vi "Compare file size of FTP to Dir on local Machine.vi"(8 "File Pattern (*.CSV .ddf)":string, 9 "Local Path to compare file sizes to FTP":path, 11 "FTP Creds":T1 {"FTP Timeout (S)" min=0 max=300 step=1}) -> (3 "Equal File Sizes":cluster{"name":string, "Equal File size":bool}[](array[cluster]))   [LabVIEW 2011]
uses:
  Controls/FTP Credintials.ctl
  <vilib>/addons/internet/NI_InternetTK_FTP_VIs.lvlib
panel:
  in  "Archive Location":path=path "C:/Archive" caption="Directory To Archive *.RAT files"
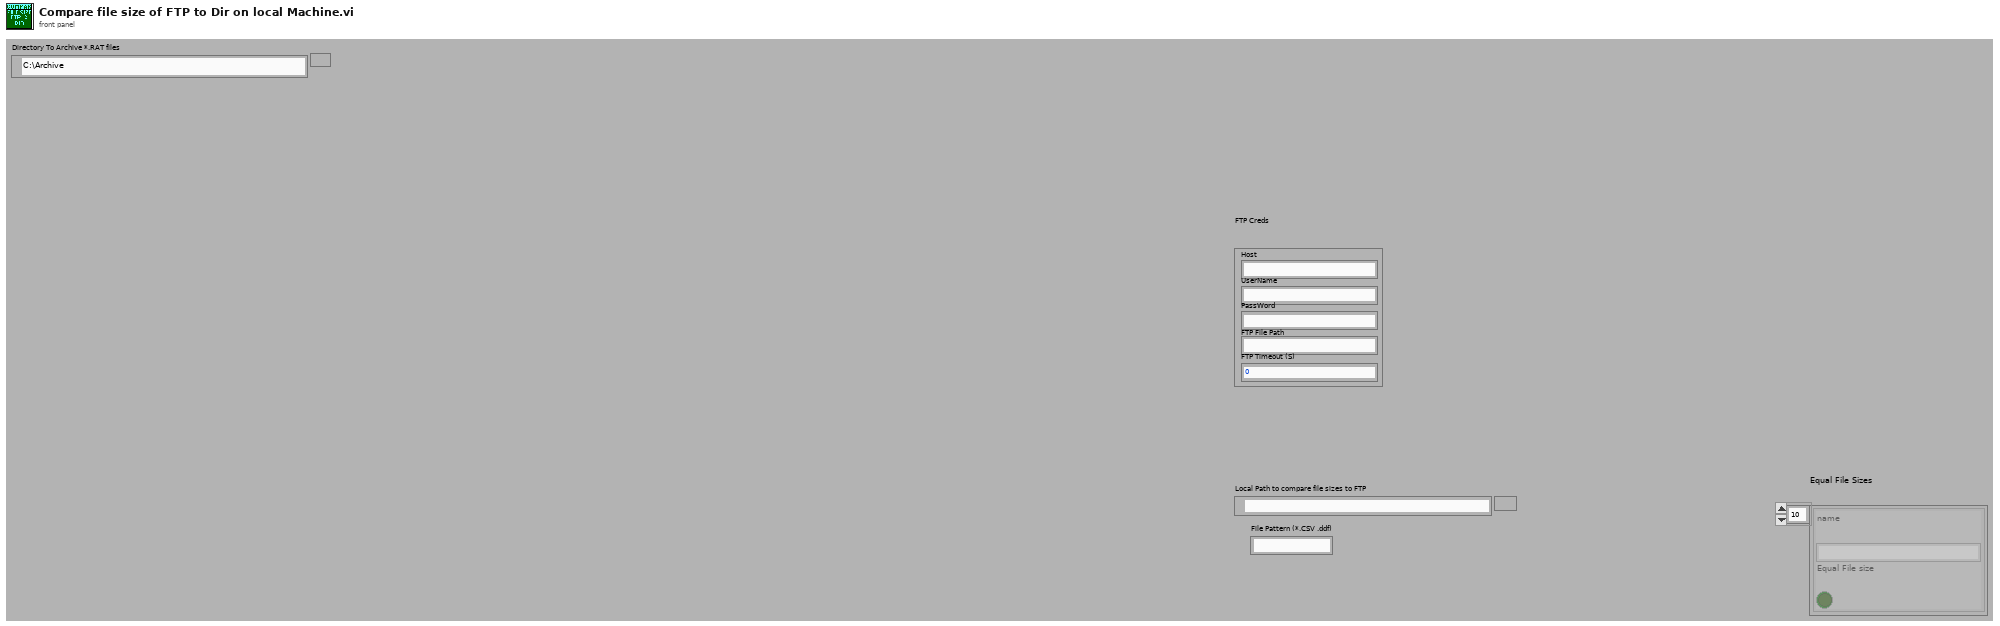
[diagram p1: front panel]
types:
  T1 = typedef "FTP Credintials.ctl" = cluster{"Host":string, "UserName":string, "PassWord":string, "FTP File Path":string, "FTP Timeout (S)":i32, "Active or Passive":bool, "ASCII or Binary":bool}
  T2 = typedef "FTP Session.ctl" = refnum<k1>
  T3 = typedef "FTP File Info.ctl" = cluster{"type":enum16{"unknown", "file", "dir", "link"}, "permissions":string, "owner":string, "group":string, "size":i32, "date":string, "name":string, "link name":string}
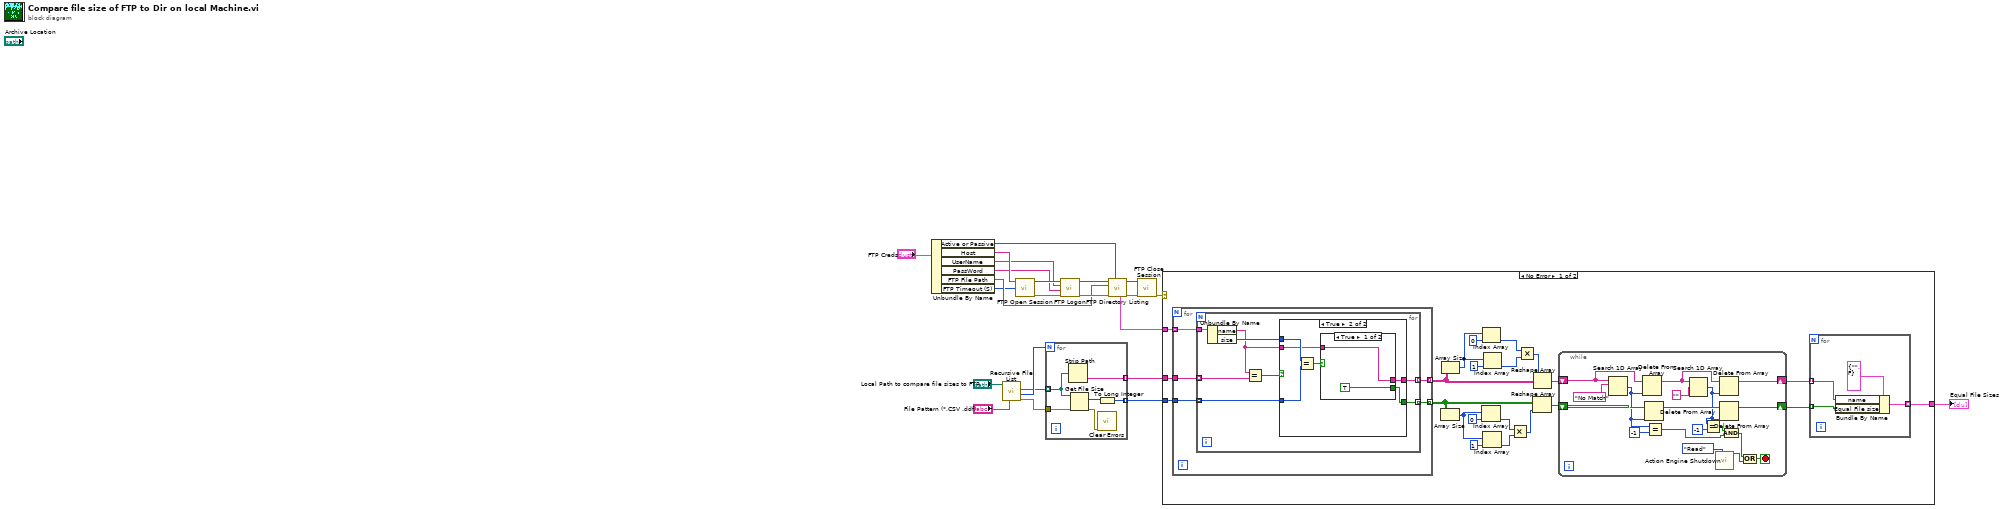
[diagram p0: block diagram]
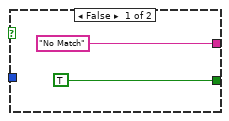
[diagram p2: hidden frame]
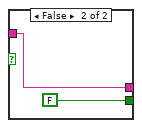
[diagram p3: hidden frame]
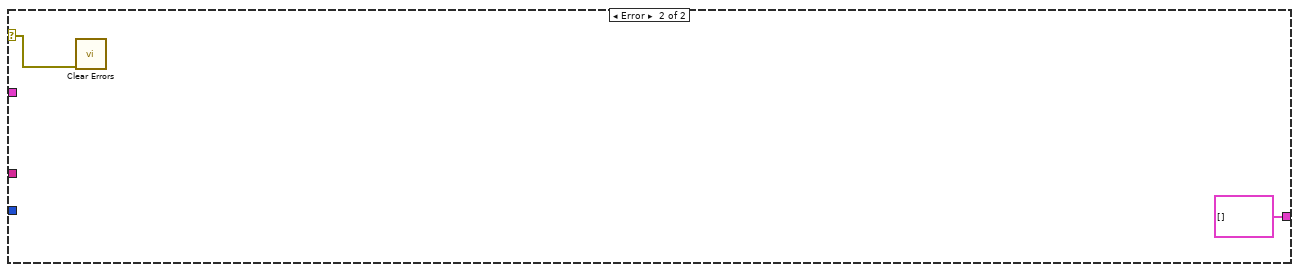
[diagram p4: hidden frame]
diagram:
  n1 = Unbundle By Name("FTP Creds") -> ("Active or Passive"=w5:bool, "Host"=w16:string, "UserName"=w15:string, "PassWord"=w14:string, "FTP File Path"=w13:string, "FTP Timeout (S)"=w2:i32)
  n2 = call <vilib>:"Recursive File List.vi"("pattern"="File Pattern (*.CSV .ddf)", "Folder Path"="Local Path to compare file sizes to FTP") -> ("error out"=w1:errorcluster, "Number of Files"=w12:i32, "All Files in Dir"=w11:path[])  [unwired: 5 in, 2 out]
  n3 = call <vilib>:"FTP Open Session.vi"("timeout ms (60000)"=w2, "address"=w16) -> ("error out"=w22:errorcluster, "ftp session"=w23:T2)  [unwired: 6 in, 2 out]
  n4 = for {
    N: w12 -> [_]
    tunnel: w11 -> [w29] mode=indexing
    tunnel: [w28] -> w8 mode=indexing
    tunnel: [w26] -> w7 mode=indexing
    tunnel: w1 -> [w25]
    n5 = Strip Path(path=w29) -> (name=w28:string)  [unwired: 1 out]
    n6 = Get File Size(file=w29, error in=w25) -> (size (in bytes)=w27:i64, 0:w24:errorcluster)  [unwired: 1 out]
    n7 = To Long Integer(number=w27) -> (32bit integer=w26:i32)
    n8 = call <vilib>:"Clear Errors.vi"("error in (no error)"=w24) -> ()  [unwired: 6 in, 1 out]
  }
  n9 = call <vilib>:"FTP Logon.vi"("error in (no error)"=w22, "password"=w14, "user"=w15, "ftp session"=w23) -> ("error out"=w20:errorcluster, "ftp session out"=w21:T2)  [unwired: 4 in, 2 out]
  n10 = call <vilib>:"FTP Directory Listing.vi"("active (T)"=w5, "error in (no error)"=w20, "directory path"=w13, "ftp session"=w21) -> ("error out"=w18:errorcluster, "ftp session out"=w19:T2, "dir list"=w9:T3[])  [unwired: 3 in, 2 out]
  n11 = call <vilib>:"FTP Close Session.vi"("error in (no error)"=w18, "ftp session"=w19) -> ("error out"=w3:errorcluster)  [unwired: 6 in, 3 out]
  n12 = case shown="No Error" w3 {
    selector: w3 -> [_ w100]
    tunnel: w9 -> [w51 _]
    tunnel: w8 -> [w50 _]
    tunnel: w7 -> [w49 _]
    tunnel: [w46 cluster{"name":string, "Equal File size":bool}[] []] -> w6
    frame No Error {
      n13 = for {
        tunnel: w51 -> [w78] mode=indexing
        tunnel: w50 -> [w77]
        tunnel: w49 -> [w76]
        tunnel: [w75] -> w32 mode=indexing
        tunnel: [w74] -> w45 mode=indexing
        n14 = for {
          tunnel: w78 -> [w86]
          tunnel: w77 -> [w84] mode=indexing
          tunnel: w76 -> [w82] mode=indexing
          tunnel: [w80] -> w74 mode=indexing
          tunnel: [w79] -> w75 mode=indexing
          n15 = Unbundle By Name(w86) -> ("name"=w81:string, "size"=w83:i32)
          n16 = Equal?(x=w81, y=w84) -> (x = y?=w85:bool)
          n17 = case shown="True" w85 {
            tunnel: w83 -> [_ w93]
            tunnel: w82 -> [_ w92]
            tunnel: w81 -> [_ w91]
            tunnel: ["No Match" ("name") w89] -> w80
            tunnel: [TRUE w90] -> w79
            frame False {
            }
            frame True {
              n18 = Equal?(x=w93, y=w92) -> (x = y?=w94:bool)
              n19 = case shown="True" w94 {
                tunnel: w91 -> [w95 w97]
                tunnel: [TRUE FALSE] -> w90
                tunnel: [w95 w97] -> w89
                frame True {
                }
                frame False {
                }
              }
            }
          }
        }
      }
      n20 = Array Size(array=w32) -> (size(s)=w35:i32[])
      n21 = Array Size(array=w45) -> (size(s)=w42:i32[])
      n22 = Index Array(array=w35, index=0) -> (element=w36:i32)
      n23 = Index Array(array=w42, index=0) -> (element=w41:i32)
      n24 = Index Array(array=w35, index=1) -> (element=w37:i32)
      n25 = Index Array(array=w42, index=1) -> (element=w40:i32)
      n26 = Multiply(x=w36, y=w37) -> (x*y=w38:i32)
      n27 = Multiply(x=w41, y=w40) -> (x*y=w39:i32)
      n28 = Reshape Array(w32, w38) -> (w30:bool[])
      n29 = Reshape Array(w45, w39) -> (w31:string[])
      n30 = while {
        shift-right: [w65] -> w48
        shift-left: w31 -> [w72]
        shift-right: [w66] -> w47
        shift-left: w30 -> [w71]
        stop <- w59 stop-if-true
        n31 = Search 1D Array(1D array=w72, element="No Match" ("name")) -> (index of element=w70:i32)  [unwired: 1 in]
        n32 = Delete From Array(array=w72, index=w70) -> (array with subset deleted=w64:string[])  [unwired: 1 in, 1 out]
        n33 = Delete From Array(array=w71, index=w70) -> (array with subset deleted=w67:bool[])  [unwired: 1 in, 1 out]
        n34 = Equal?(x=w70, y=-1) -> (x = y?=w60:bool)
        n35 = Search 1D Array(1D array=w64, element="" ("name")) -> (index of element=w62:i32)  [unwired: 1 in]
        n36 = Equal?(x=w62, y=-1) -> (x = y?=w61:bool)
        n37 = call "Action Engine Shutdown.vi"("Shutdown"=enum16{"Write", "Read"}."Read") -> ("Shutdown"=w56:bool)  [unwired: 9 in, 1 out]
        n38 = Delete From Array(array=w64, index=w62) -> (array with subset deleted=w65:string[])  [unwired: 1 in, 1 out]
        n39 = Delete From Array(array=w67, index=w62) -> (array with subset deleted=w66:bool[])  [unwired: 1 in, 1 out]
        n40 = And(x=w61, y=w60) -> (x .and. y?=w58:bool)
        n41 = Or(x=w58, y=w56) -> (x .or. y?=w59:bool)
      }
      n42 = for {
        tunnel: w48 -> [w54] mode=indexing
        tunnel: w47 -> [w53] mode=indexing
        tunnel: [w52] -> w46 mode=indexing
        n43 = Bundle By Name(cluster=cluster{"name":string, "Equal File size":bool} {"name"="", "Equal File size"=FALSE} ("input cluster"), "name"=w54, "Equal File size"=w53) -> (w52:cluster{"name":string, "Equal File size":bool})
      }
    }
    frame Error {
      n44 = call <vilib>:"Clear Errors.vi"("error in (no error)"=w100) -> ()  [unwired: 6 in, 1 out]
    }
  }
  "Equal File Sizes" <- w6
